vi "Set Default Values.vi"(10 "Default Values in":variant[](array[variant]), 11 "VI in":refnum<vi>) -> ()   [LabVIEW 2013]
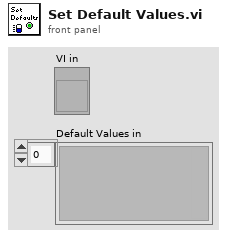
[diagram p1: front panel]
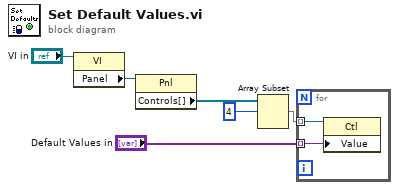
[diagram p0: block diagram]
diagram:
  n1 = property class="VI"(reference="VI in") -> ("Panel"=w5:refnum<vi>)  [unwired: 1 in, 2 out]
  n2 = property class="Pnl"(reference=w5) -> ("Controls[]"=w3:refnum<vi>[])  [unwired: 1 in, 2 out]
  n3 = Array Subset(array=w3, index=4) -> (w1:refnum<vi>[])  [unwired: 1 in]
  n4 = for {
    tunnel: w1 -> [w8] mode=indexing
    tunnel: "Default Values in" -> [w7] mode=indexing
    n5 = property class="Ctl"(reference=w8, "Value"=w7) -> ()  [unwired: 1 in, 2 out]
  }
